vi "FTW-CodeGen-Image-Subset.vi"(1 "Left":i32 format="%dpx", 2 "24-bit Image":T1, 4 "Height":i32 format="%dpx", 5 "Top":i32 format="%dpx", 8 "Width":i32 format="%dpx") -> (7 "Image subset":T1)   [LabVIEW 2015]
panel:
  # "Inputs"
  # "Outputs"
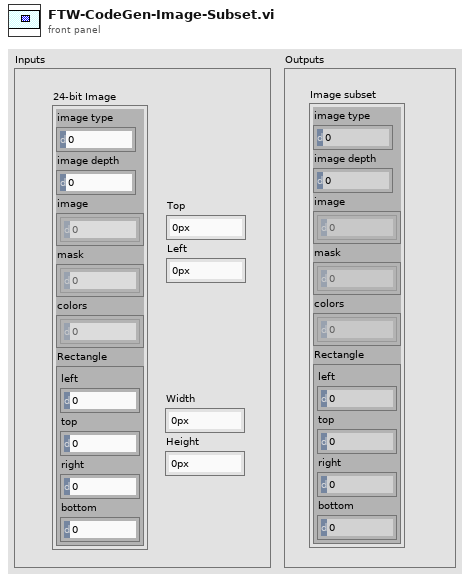
[diagram p1: front panel]
types:
  T1 = cluster{"image type":i32, "image depth":i32, "image":u8[], "mask":u8[], "colors":u32[], "Rectangle":cluster{"left":i16, "top":i16, "right":i16, "bottom":i16}}
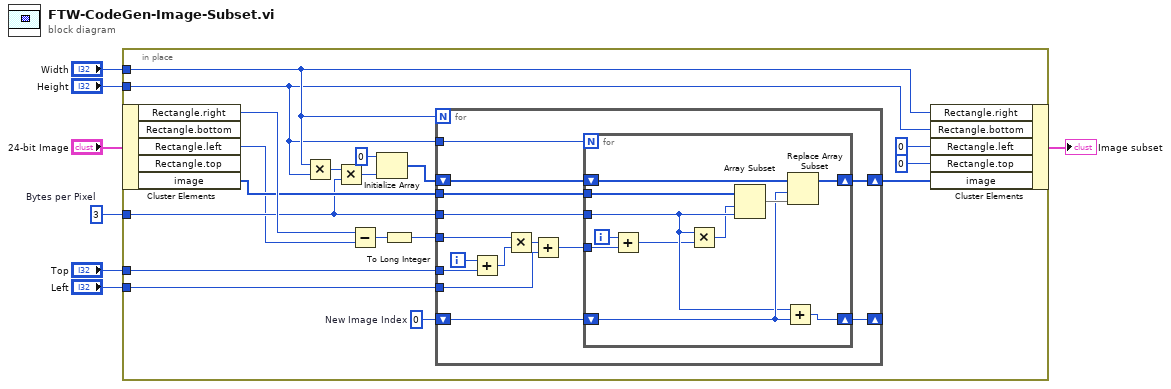
[diagram p0: block diagram]
diagram:
  w7 = 3  # Bytes per Pixel
  n1 = in-place {
    in-place-border: "Top" -> [w22]
    in-place-border: "Left" -> [w21]
    in-place-border: "Width" -> [w16]
    in-place-border: "Height" -> [w15]
    in-place-border: w7 -> [w12]
    w23 = 0  # New Image Index
    n2 = in-place-cluster #1("24-bit Image") -> ("Rectangle.right"=w20:i16, "Rectangle.left"=w8:i16, "image"=w13:u8[])  [unwired: 2 out]
    n3 = Multiply(x=w16, y=w15) -> (x*y=w18:i32)
    n4 = Multiply(x=w18, y=w12) -> (x*y=w17:i32)
    n5 = Subtract(x=w20, y=w8) -> (x-y=w19:i16)
    n6 = Initialize Array(u8 0 ("element"), w17) -> (w25:u8[])
    n7 = To Long Integer(number=w19) -> (32bit integer=w11:i32)
    n8 = for {
      N: w16 -> [_]
      tunnel: w13 -> [w39]
      tunnel: w15 -> [w38]
      shift-right: [w36] -> w14
      shift-left: w25 -> [w37]
      shift-right: [w34] -> _
      shift-left: w23 -> [w35]
      tunnel: w12 -> [w32]
      tunnel: w22 -> [w33]
      tunnel: w21 -> [w27]
      tunnel: w11 -> [w30]
      i -> [w31]
      n9 = Add(x=w31, y=w33) -> (x+y=w29:i32)
      n10 = Multiply(x=w30, y=w29) -> (x*y=w28:i32)
      n11 = Add(x=w28, y=w27) -> (x+y=w26:i32)
      n12 = for {
        N: w38 -> [_]
        tunnel: w39 -> [w48]
        shift-right: [w49] -> w36
        shift-left: w37 -> [w50]
        shift-right: [w46] -> w34
        shift-left: w35 -> [w45]
        tunnel: w26 -> [w44]
        tunnel: w32 -> [w42]
        i -> [w43]
        n13 = Add(x=w43, y=w44) -> (x+y=w40:i32)
        n14 = Multiply(x=w42, y=w40) -> (x*y=w41:i32)
        n15 = Array Subset(array=w48, index=w41, length=w42) -> (w47:u8[])
        n16 = Add(x=w42, y=w45) -> (x+y=w46:i32)
        n17 = Replace Array Subset(array=w50, new element=w47, index=w45) -> (w49:u8[])
      }
    }
    n18 = in-place-cluster #1("Rectangle.right"=w16, "Rectangle.bottom"=w15, "Rectangle.left"=i16 0, "Rectangle.top"=i16 0, "image"=w14) -> (→"Image subset":T1)
  }
